vi "Status.vi"(8 "error in (no error)":errorcluster, 10 "Internal?":bool, 11 "Julabo FP-50 Settings":T1={"VISA resource name"="", "Simulated?"=FALSE, "Pump Power"=2} {"Pump Power" min=0 max=8 step=1}) -> (0 "error out":errorcluster, 1 "Connection Error":bool, 2 "Running":bool, 3 "Julabo FP-50 Settings":T1={"VISA resource name"="", "Simulated?"=FALSE, "Pump Power"=2} {"Pump Power" min=0 max=8 step=1}, 4 "Temp":dbl, 6 "Pumpstage (out)":u8)   [LabVIEW 2018, in "Julabo Type FP-50 TCU.lvlib"]
uses:
  Julabo Type FP-50 TCU.lvlib
  Julabo FP-50 Settings.ctl
  Third Party Drivers/Julabo Type 1/JULABO DeviceDriver/JULABO DeviceDriver.lvlib
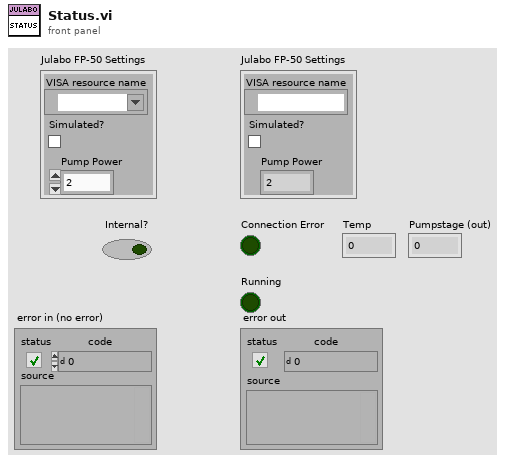
[diagram p1: front panel]
types:
  T1 = typedef "Julabo Type FP-50 TCU.lvlib/Julabo FP-50 Settings.ctl" = cluster{"VISA resource name":refnum<visa-resource-name>, "Simulated?":bool, "Pump Power":i32}
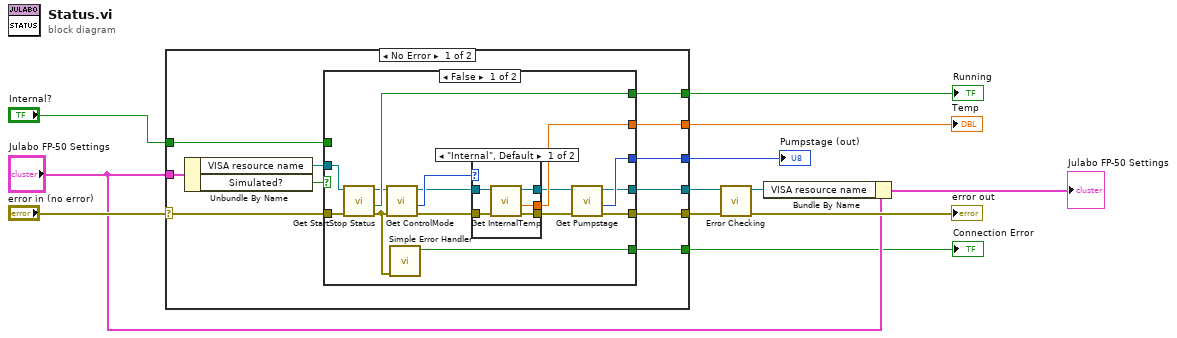
[diagram p0: block diagram]
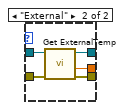
[diagram p2: hidden frame]
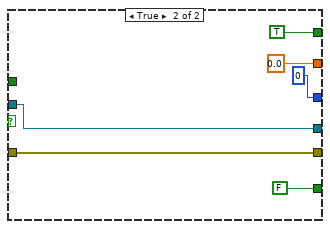
[diagram p3: hidden frame]
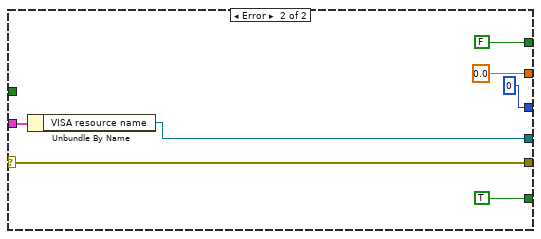
[diagram p4: hidden frame]
diagram:
  n1 = case shown="No Error" "error in (no error)" {
    selector: "error in (no error)" -> [w23 w61]
    tunnel: "Julabo FP-50 Settings" -> [w21 w60]
    tunnel: [w22 w61] -> w10
    tunnel: [w19 w59] -> w11
    tunnel: [w17 TRUE] -> w5
    tunnel: [w16 FALSE] -> w4
    tunnel: "Internal?" -> [w15 _]
    tunnel: [w14 0.0 ("InternalTemp (out)")] -> w2
    tunnel: [w13 u8 0 ("Pumpstage (out)")] -> w1
    frame No Error {
      n2 = Unbundle By Name(w21) -> ("VISA resource name"=w20:refnum<visa-resource-name>, "Simulated?"=w18:bool)
      n3 = case shown="False" w18 {
        tunnel: w23 -> [w37 w54]
        tunnel: [w24 w54] -> w22
        tunnel: [w26 w53] -> w19
        tunnel: w20 -> [w38 w53]
        tunnel: [w35 FALSE] -> w17
        tunnel: [w36 TRUE] -> w16
        tunnel: w15 -> [_ _]
        tunnel: [w34 0.0 ("InternalTemp (out)")] -> w14
        tunnel: [w28 u8 0 ("Pumpstage (out)")] -> w13
        frame False {
          n4 = call "Get StartStop Status.vi"("error in"=w37, "VISA resource name in"=w38) -> ("error out"=w32:errorcluster, "Status"=w36:bool, "VISA resource name out"=w33:refnum<visa-resource-name>)  [unwired: 7 in]
          n5 = call "Get ControlMode.vi"("error in"=w32, "VISA resource name in"=w33) -> ("error out"=w29:errorcluster, "Control (out)"=w31:enum16{"Internal", "External"}, "VISA resource name out"=w30:refnum<visa-resource-name>)  [unwired: 7 in]
          n6 = call <vilib>:"Simple Error Handler.vi"("error in (no error)"=w32) -> ("error?"=w35:bool)  [unwired: 4 in, 4 out]
          n7 = case shown="\"Internal\", Default" w31 {
            tunnel: w30 -> [w43 w48]
            tunnel: w29 -> [w42 w47]
            tunnel: [w41 w45] -> w27
            tunnel: [w40 w46] -> w25
            tunnel: [w39 w44] -> w34
            frame "Internal", Default {
              n8 = call "Get InternalTemp.vi"("error in (no error)"=w42, "VISA resource name"=w43) -> ("error out"=w40:errorcluster, "InternalTemp (out)"=w39:dbl, "VISA resource name out"=w41:refnum<visa-resource-name>)  [unwired: 7 in]
            }
            frame "External" {
              n9 = call "Get ExternalTemp.vi"("error in (no error)"=w47, "VISA resource name"=w48) -> ("error out"=w46:errorcluster, "ExternalTemp (out)"=w44:dbl, "VISA resource name out"=w45:refnum<visa-resource-name>)  [unwired: 6 in, 1 out]
            }
          }
          n10 = call "Get Pumpstage.vi"("error in (no error)"=w25, "VISA resource name"=w27) -> ("error out"=w24:errorcluster, "Pumpstage (out)"=w28:u8, "VISA resource name out"=w26:refnum<visa-resource-name>)  [unwired: 7 in]
        }
        frame True {
        }
      }
    }
    frame Error {
      n11 = Unbundle By Name(w60) -> ("VISA resource name"=w59:refnum<visa-resource-name>)
    }
  }
  "Connection Error" <- w5
  "Running" <- w4
  "Temp" <- w2
  "Pumpstage (out)" <- w1
  n12 = call "Error Checking.vi"("error in (no error)"=w10, "VISA resource name"=w11) -> ("error out"=→"error out":errorcluster, "VISA resource name"=w8:refnum<visa-resource-name>)  [unwired: 7 in, 1 out]
  n13 = Bundle By Name(cluster="Julabo FP-50 Settings", "VISA resource name"=w8) -> (→"Julabo FP-50 Settings":T1)
